vi "Manual Intake Control.vi"   [LabVIEW 2015]
uses:
  Robot Global Data.vi
types:
  T1 = typedef "Dashboard Control Data.ctl" = cluster{"Auton Loops":dbl, "Shooter Presets":T2, "Encoder Control":T4, "Intake Command CLuster ":cluster{"Intake Speed":dbl, "HP Load Speed":dbl, "Turn Out Speed":dbl, "Turn In Speed":dbl, "Unload Speed":dbl}}
  T2 = typedef "Shooter Presets.ctl" = cluster{"Batter Shot":T3, "Low Bar Curve Shot":T3, "Deep Middle Shot":T3, "Manual Shot":T3}
  T3 = typedef "Shot Presets.ctl" = cluster{"Left Wheel RPM":dbl, "Right Wheel RPM":dbl}
  T4 = typedef "Encoder Control.ctl" = cluster{"Right Tick Constat":dbl, "Left Tick Constant":dbl, "Reset?":bool, "Y Dist":cluster{"PID gains":cluster{"proportional gain (Kc)":dbl, "integral time (Ti, min)":dbl, "derivative time (Td<min)":dbl}}, "Y Stop Thresh":dbl, "Y Stop Speed":dbl}
  T5 = cluster{"Intake Speed":dbl, "HP Load Speed":dbl, "Turn Out Speed":dbl, "Turn In Speed":dbl, "Unload Speed":dbl}
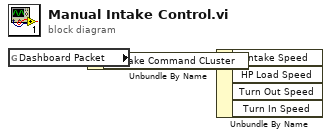
[diagram p0: block diagram]
diagram:
  n1 = global read "Robot Global Data.vi" "Dashboard Packet"() -> (w2:T1)
  n2 = Unbundle By Name(w2) -> ("Intake Command CLuster"=w1:T5)
  n3 = Unbundle By Name(w1) -> ()  [unwired: 4 out]
